vi "pulse_generator_multiheater_refnum_switch_value_getter.vi"(0 "On/Off Refnums":refnum<vi>[](array[refnum])) -> (1 "Analog[0-10]":dbl[](array[numeric]) format="%#_13g", 2 "Digital":bool[](array[boolean]))   [LabVIEW 2017]
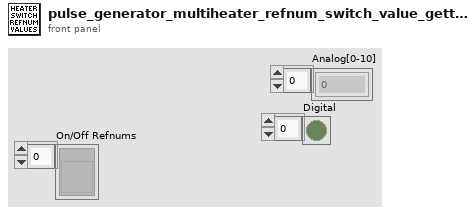
[diagram p1: front panel]
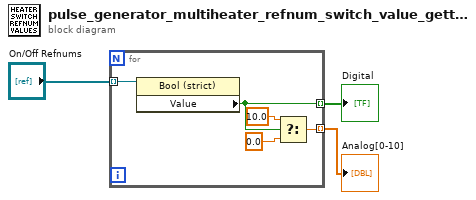
[diagram p0: block diagram]
diagram:
  n1 = for {
    tunnel: "On/Off Refnums" -> [w8] mode=indexing
    tunnel: [w5] -> w3 mode=indexing
    tunnel: [w4] -> w2 mode=indexing
    n2 = property class="Bool (strict)"(reference=w8) -> ("Value"=w4:bool)  [unwired: 1 in, 2 out]
    n3 = Select(t=10.0, s=w4, f=0.0) -> (s? t:f=w5:dbl)
  }
  "Analog[0-10]" <- w3
  "Digital" <- w2
